vi "filecopy.vi"() -> ()   [LabVIEW 2014]
panel:
  in  "Target Path":path
  in  "Source Path":path
  in  "stop":bool
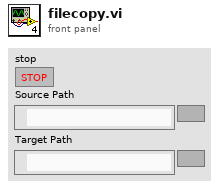
[diagram p1: front panel]
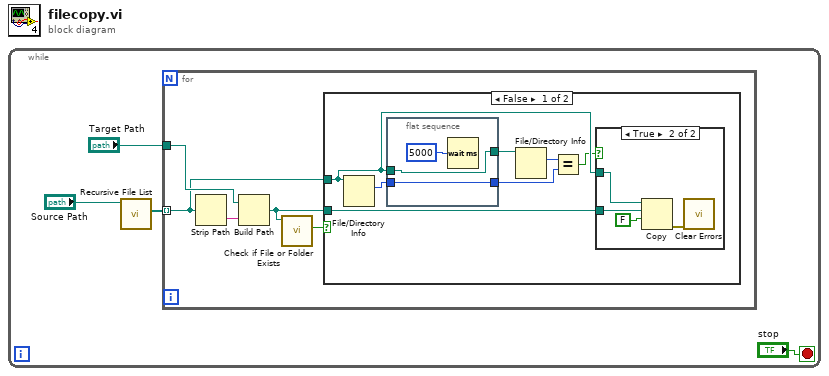
[diagram p0: block diagram]
diagram:
  n1 = while {
    stop <- "stop" stop-if-true
    n2 = call <vilib>:"Recursive File List.vi"("Folder Path"="Source Path") -> ("All Files in Dir"=w2:path[])  [unwired: 6 in, 4 out]
    n3 = for {
      tunnel: w2 -> [w5] mode=indexing
      tunnel: "Target Path" -> [w8]
      n4 = Strip Path(path=w5) -> (name=w6:string)  [unwired: 1 out]
      n5 = Build Path(base path=w8, name or relative path=w6) -> (appended path=w7:path)
      n6 = call <vilib>:"Check if File or Folder Exists.vi"("path"=w7) -> ("file or folder exists?"=w9:bool)  [unwired: 8 in, 2 out]
      n7 = case shown="False" w9 {
        tunnel: w7 -> [w16 _]
        tunnel: w5 -> [w13 _]
        frame False {
          n8 = File/Directory Info(path=w13) -> (size=w15:i64)  [unwired: 1 in, 6 out]
          n9 = flat-sequence {
            tunnel: w15 -> [w17]
            tunnel: [w18] -> w14
            tunnel: w13 -> [w18]
            tunnel: [w17] -> w11
            frame #0 {
              n10 = Wait (ms)(milliseconds to wait=u32 5000) -> ()  [unwired: 1 out]
            }
          }
          n11 = File/Directory Info(path=w14) -> (size=w12:i64)  [unwired: 1 in, 6 out]
          n12 = Equal?(x=w12, y=w11) -> (x = y?=w10:bool)
          n13 = case shown="True" w10 {
            tunnel: w16 -> [_ w21]
            tunnel: w13 -> [_ w20]
            frame False {
            }
            frame True {
              n14 = Copy(9:FALSE ("overwrite (F)"), 10:w21, 11:w20) -> (0:w22:errorcluster)  [unwired: 2 in, 2 out]
              n15 = call <vilib>:"Clear Errors.vi"("error in (no error)"=w22) -> ()  [unwired: 5 in, 2 out]
            }
          }
        }
        frame True {
        }
      }
    }
  }
